vi "testFlattenArrayAtRootLevel.vi"(8 "error in (no error)":errorcluster, 11 "reference in":refnum<class "EasyXMLTest.lvclass">) -> (0 "error out":errorcluster, 3 "reference in":refnum<class "EasyXMLTest.lvclass">)   [LabVIEW 2011, in "EasyXMLTest.lvclass"]
uses:
  EasyXMLTest.lvclass
panel:
  out "Generated XML String":string
  out "XML String":string
  out "Input Data":variant
  out "Produced Data":variant
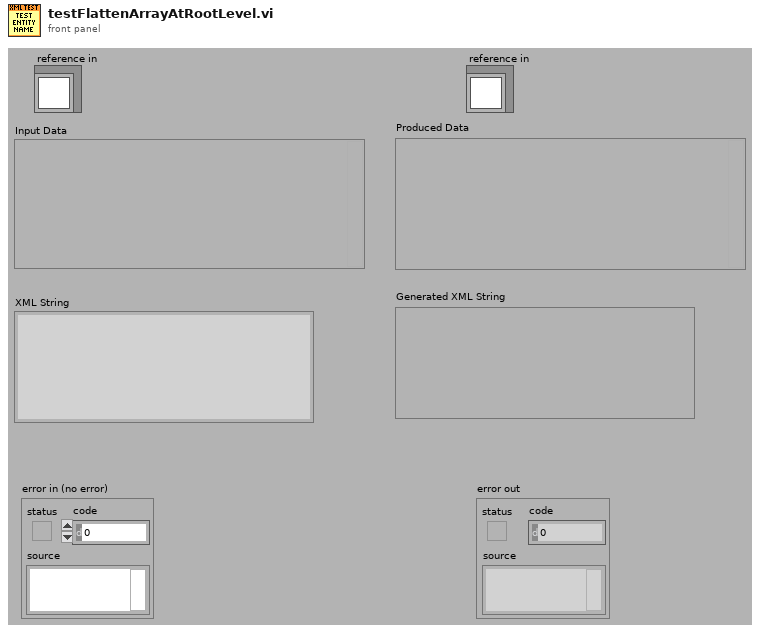
[diagram p1: front panel]
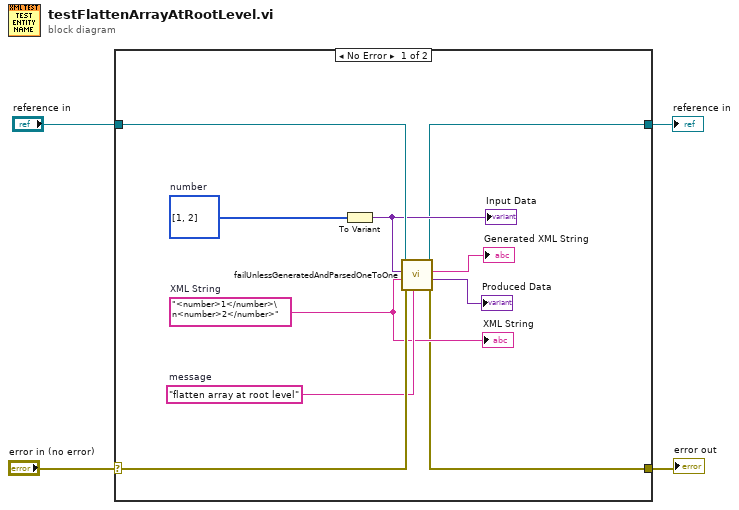
[diagram p0: block diagram]
diagram:
  n1 = case shown="No Error" "error in (no error)" {
    selector: "error in (no error)" -> [w13 w16]
    tunnel: [w6 w16] -> w3
    tunnel: [w5 w15] -> w1
    tunnel: "reference in" -> [w14 w15]
    frame No Error {
      w10 = i32[] [1, 2]  # number
      w12 = "flatten array at root level"  # message
      w11 = "<number>1</number>\n<number>2</number>"  # XML String
      n2 = To Variant(anything=w10) -> (Variant=w8:variant)
      "Input Data" <- w8
      n3 = call "failUnlessGeneratedAndParsedOneToOne.vi"("message (\"\")"=w12, "error in"=w13, "XML String"=w11, "Data"=w8, "EasyXMLTest in"=w14) -> ("error out"=w6:errorcluster, "Produced Data"=→"Produced Data":variant, "Generated XML String"=→"Generated XML String":string, "EasyXMLTest out"=w5:refnum<class "EasyXMLTest.lvclass">)  [unwired: 3 in]
      "XML String" <- w11
    }
    frame Error {
    }
  }
  "error out" <- w3
  "reference in" <- w1
